vi "TRA server.vi"() -> ()   [LabVIEW 2011]
uses:
  <vilib>/regexp/Match Regular Expression.xnode
panel:
  out "SEND ME TO TRA":string
  in  "Active":bool=TRUE
  out "stopCmd":bool
  out "stopAnswer":string
  out "sema free":bool
  out "Answer Q":refnum<queue>
  out "CmdID":string
  out "in Progress":bool=TRUE
  out "Diode":bool
  in  "STOP":bool
  in  "Tab Control":enum32{"Main", "Config", "Error", "History"}(tab)=enum."Config"
  out "time between two execution":u32
  out "answer":string
  in  "reset array":bool=TRUE
  out "ExecutedCmd":T1(array[cluster])
  out "ConnectArray":T2(array[cluster])
  in  "Picopad Name":string="TRA1"
  in  "Mode GPIB / VISA":bool
  out "NameComment":string
  in  "Port":i32=63430
  out "DevicesConnected":string[][](array[string])
  out "CmdInProgress":T3(array[cluster])
  out "A Q error":errorcluster
  out "tcp error":errorcluster
  out "History":T1(array[cluster])
  out "stopOc":refnum<k4>
  out "semaphore":T4
  out "timer in":u32
  out "Execute time in":u32
  out "Cmd received":string
  # "Server info:"
  # "Don't wire GPIB and VISA on the same time, VISA will be non reliable"
  # "slot3"
  # "slot5"
  # "Slot1"
  # "slot2"
  # "slot4"
  # "connector1"
  # "connector2"
  # "connector3"
  # "connector4"
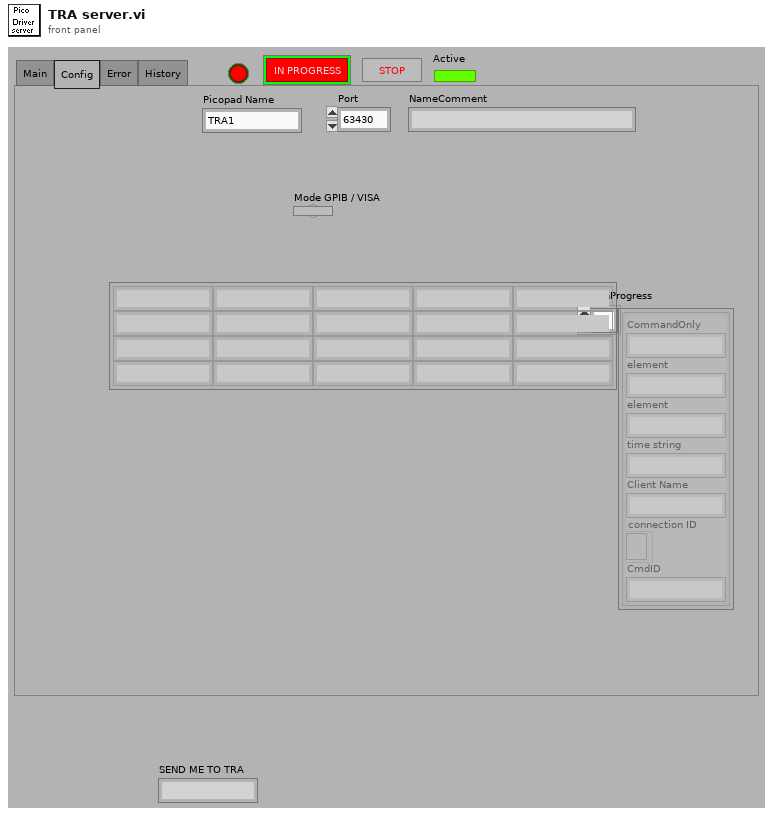
[diagram p1: front panel]
types:
  T1 = cluster{"CommandOnly":string, "status":string, "duration":string, "date":string, "Client Name":string, "connection ID":refnum<k5>, "CmdID":string}[]
  T2 = cluster{"connection ID":refnum<k5>, string, errorcluster}[]
  T3 = cluster{"CommandOnly":string, "element":string, "element":string, "time string":string, "Client Name":string, "connection ID":refnum<k5>, "CmdID":string}[]
  T4 = typedef "Semaphore RefNum" = refnum<k1>
  T5 = cluster{"CommandOnly":string, "element":string, "element":string, "time string":string, "Client Name":string, "connection ID":refnum<k5>, "CmdID":string}
  T6 = cluster{"CommandOnly":string, "status":string, "duration":string, "date":string, "Client Name":string, "connection ID":refnum<k5>, "CmdID":string}
  T7 = cluster{"CommandOnly":string, "status":string, "element":string, "time string":string, "Client Name":string, "connection ID":refnum<k5>, "CmdID":string}
  T8 = cluster{"CommandOnly":string, "status":string, "element":string, "time string":string, "Client Name":string, "connection ID":refnum<k5>, "CmdID":string}[]
  T9 = cluster{"connection ID":refnum<k5>, "remote address":string, "warning out":errorcluster}
  T10 = cluster{"connection ID":refnum<k5>, "remote address":string, "warning out":errorcluster}[]
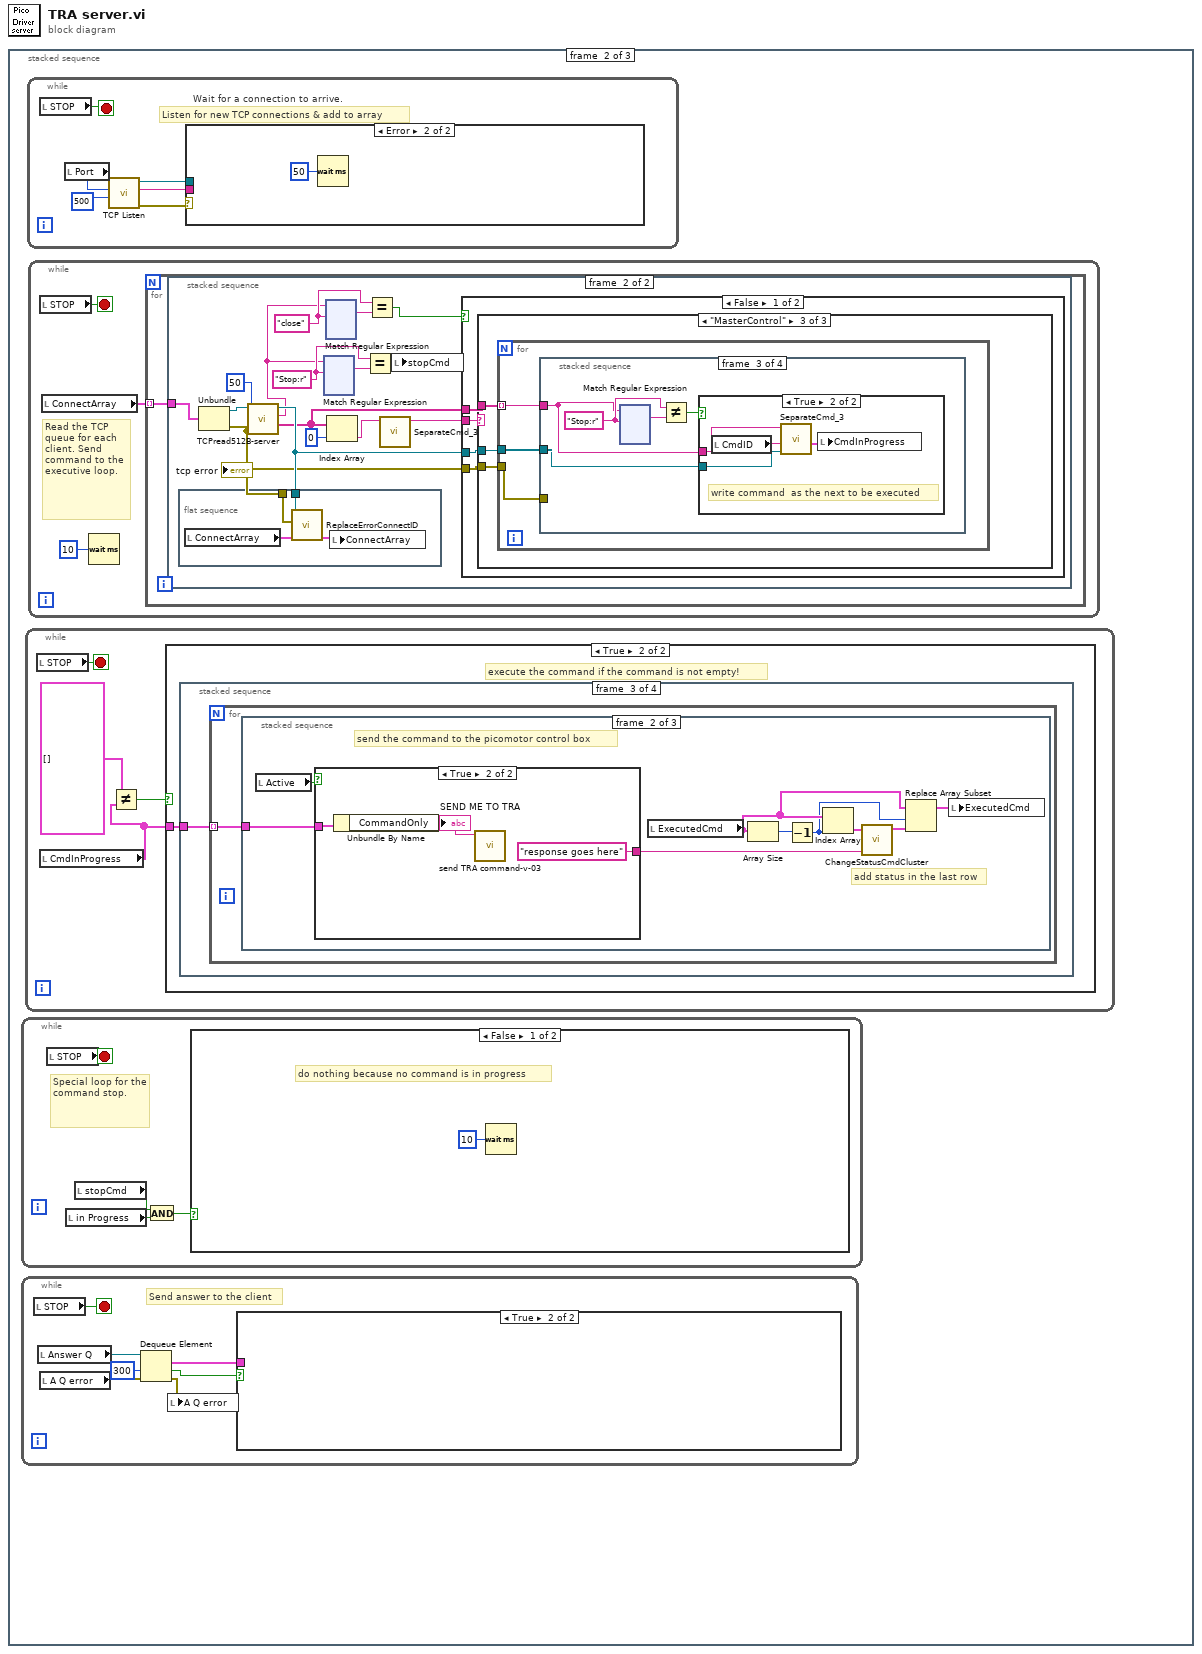
[diagram p0: block diagram]
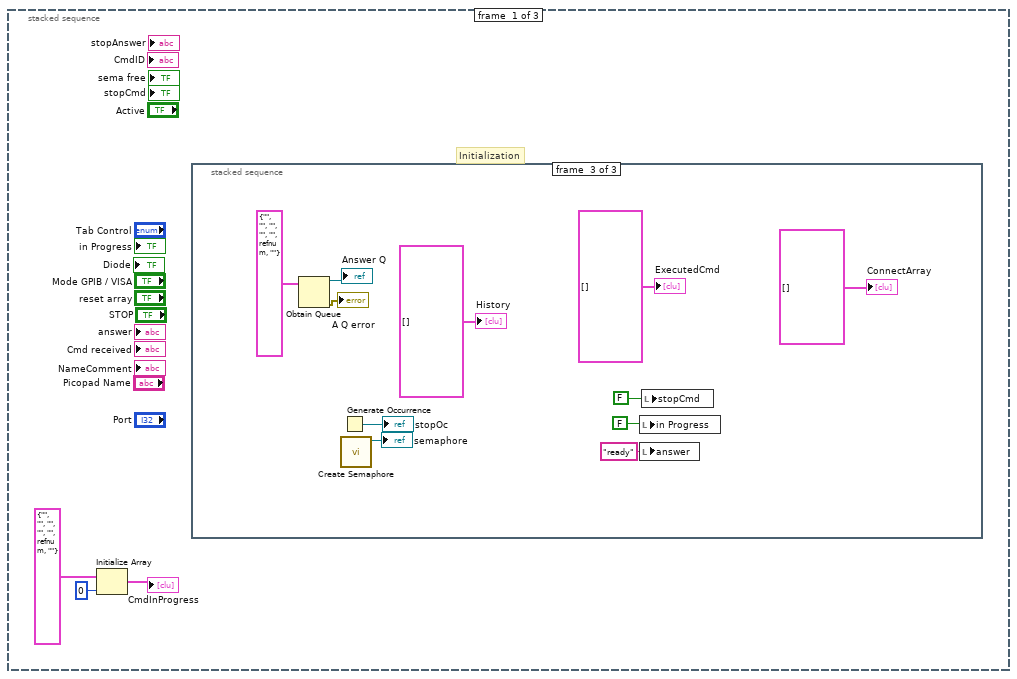
[diagram p2: hidden frame]
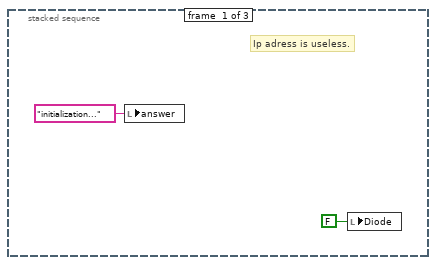
[diagram p3: hidden frame]
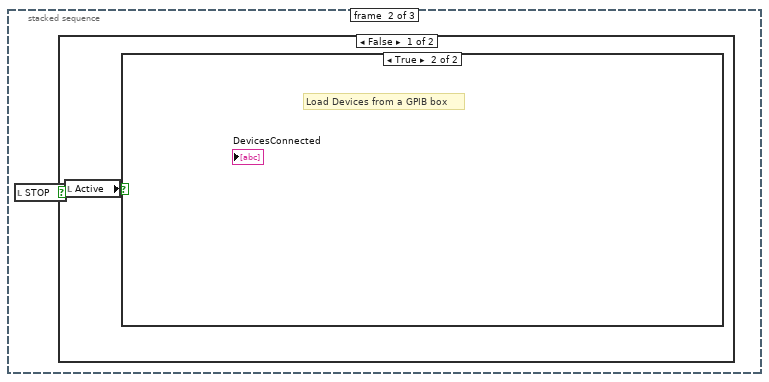
[diagram p4: hidden frame]
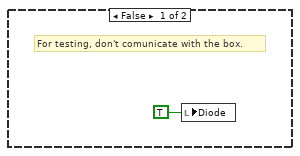
[diagram p5: hidden frame]
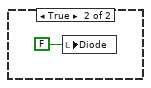
[diagram p6: hidden frame]
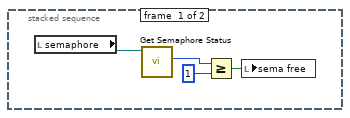
[diagram p7: hidden frame]
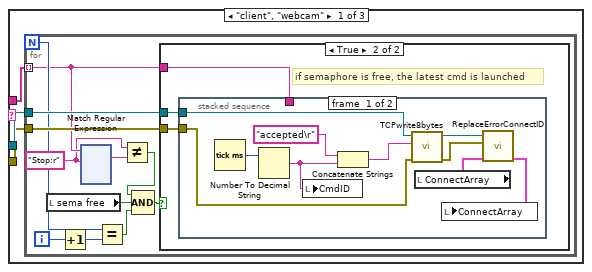
[diagram p8: hidden frame]
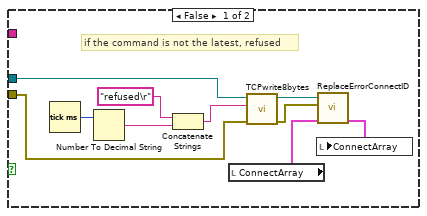
[diagram p9: hidden frame]
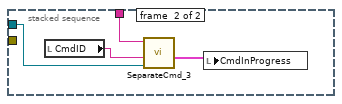
[diagram p10: hidden frame]
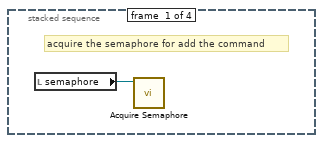
[diagram p12: hidden frame]
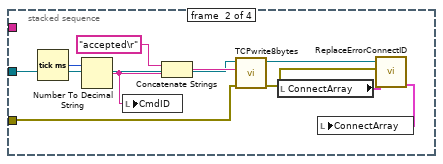
[diagram p13: hidden frame]
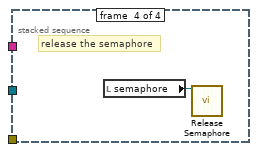
[diagram p15: hidden frame]
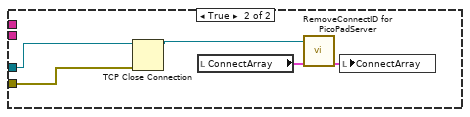
[diagram p16: hidden frame]
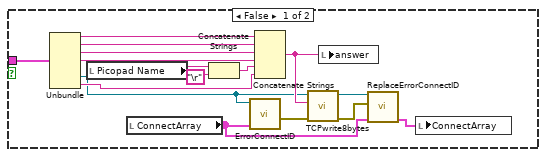
[diagram p17: hidden frame]
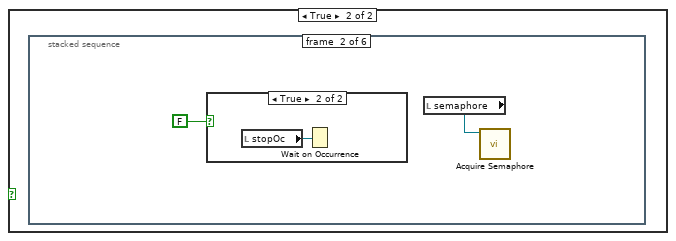
[diagram p18: hidden frame]
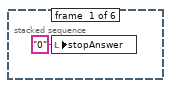
[diagram p19: hidden frame]
diagram:
  n1 = stacked-sequence {
    frame #0 {
      # "Initialization"
      n2 = Initialize Array(T5 {"CommandOnly"="", "element"="", "element"="", "time string"="", "Client Name"="", "connection ID"=refnum, "CmdID"=""} ("CmdInProgress"), 0 ("dimension size")) -> (→"CmdInProgress":T3)
      n3 = stacked-sequence {
        frame #0 {
          # "Ip adress is useless."
          n4 = local write "answer"("initialization..." ("answer")) -> ()
          n5 = local write "Diode"(FALSE ("Diode")) -> ()
        }
        frame #1 {
          n6 = local read "STOP"() -> (w6:bool)
          n7 = case shown="False" w6 {
            frame False {
              n8 = local read "Active"() -> (w7:bool)
              n9 = case shown="True" w7 {
                frame False {
                  # "For testing, don't comunicate with the box."
                  n10 = local write "Diode"(TRUE ("Diode")) -> ()
                }
                frame True {
                  # "Load Devices from a GPIB box"
                }
              }
            }
            frame True {
              n11 = local write "Diode"(FALSE ("Diode")) -> ()
            }
          }
        }
        frame #2 {
          n12 = Obtain Queue(element data type=T5 {"CommandOnly"="", "element"="", "element"="", "time string"="", "Client Name"="", "connection ID"=refnum, "CmdID"=""} ("CmdCluster 2")) -> (queue out=→"Answer Q":refnum<queue>, error out=→"A Q error":errorcluster)  [unwired: 3 in, 2 out]
          n13 = Generate Occurrence() -> (→"stopOc":refnum<k4>)
          n14 = call <vilib>:"Create Semaphore.vi"() -> ("semaphore"=→"semaphore":T4)  [unwired: 2 in, 5 out]
          n15 = local write "in Progress"(FALSE ("in Progress")) -> ()
          n16 = local write "answer"("ready" ("answer")) -> ()
          n17 = local write "stopCmd"(FALSE ("stopCmd")) -> ()
          "ConnectArray" <- T2 []
          "ExecutedCmd" <- T3 []
          "History" <- T3 []
        }
      }
    }
    frame #1 {
      n18 = while {
        stop <- w597 stop-if-true
        # "Special loop for the command stop."
        n19 = local read "STOP"() -> (w597:bool)
        n20 = local read "in Progress"() -> (w596:bool)
        n21 = local read "stopCmd"() -> (w594:bool)
        n22 = And(x=w594, y=w596) -> (x .and. y?=w595:bool)
        n23 = case shown="False" w595 {
          frame False {
            # "do nothing because no command is in progress"
            n24 = Wait (ms)(milliseconds to wait=u32 10) -> ()  [unwired: 1 out]
          }
          frame True {
            n25 = stacked-sequence {
              frame #0 {
                n26 = local write "stopAnswer"("0" ("stopAnswer")) -> ()
              }
              frame #1 {
                n27 = case shown="True" FALSE {
                  frame False {
                  }
                  frame True {
                    n28 = local read "stopOc"() -> (w602:refnum<k4>)
                    n29 = Wait on Occurrence(2:w602) -> ()  [unwired: 3 out]
                  }
                }
                n30 = local read "semaphore"() -> (w600:T4)
                n31 = call <vilib>:"Acquire Semaphore.vi"("semaphore"=w600) -> ()  [unwired: 2 in, 5 out]
              }
              frame #2 {
                # "send answer to the command client"
                # "add status in the last row"
                n32 = local read "stopAnswer"() -> (w604:string)
                n33 = xnode "Match Regular Expression"("input string"=w604, "regular expression"="0" ("y")) -> ("whole match"=w617:string)  [unwired: 2 in, 6 out]
                n34 = local read "ExecutedCmd"() -> (w607:T1)
                n35 = Equal?(x=w617, y="0") -> (x = y?=w618:bool)
                n36 = Select(t="aborted\r", s=w618, f=w604) -> (s? t:f=w609:string)
                n37 = Array Size(array=w607) -> (size(s)=w606:i32)
                n38 = Decrement(x=w606) -> (x-1=w605:i32)
                n39 = Index Array(array=w607, index=w605) -> (element=w611:T6)
                n40 = call "ChangeStatusCmdCluster.vi"("status"=w609, "CmdClusterIN"=w611) -> ("CmdClusterOUT"=w608:T7)  [unwired: 9 out]
                n41 = Replace Array Subset(array=w607, new element=w608, index=w605) -> (w610:T1)
                n42 = local write "ExecutedCmd"(w610) -> ()
                n43 = local read "Answer Q"() -> (w615:refnum<queue>)
                n44 = local read "A Q error"() -> (w614:errorcluster)
                n45 = Enqueue Element(queue=w615, element=w608, error in (no error)=w614) -> (error out=w603:errorcluster)  [unwired: 3 out]
                n46 = local write "A Q error"(w603) -> ()
              }
              frame #3 {
                n47 = local read "ConnectArray"() -> (w731:T2)
                n48 = for {
                  tunnel: w731 -> [w737] mode=indexing
                  tunnel: "A client sent a stop command." -> [w733]
                  n49 = Unbundle(w737) -> ("connection ID"=w736:refnum<k5>, w734:errorcluster)  [unwired: 1 out]
                  n50 = call "TCPwrite8bytes.vi"("Error in"=w734, "Cmd In"=w733, "connection ID in"=w736) -> ("Error out"=w732:errorcluster, "connection ID out"=w735:refnum<k5>)  [unwired: 7 out]
                  n51 = local read "ConnectArray"() -> (w739:T2)
                  n52 = call "ReplaceErrorConnectID.vi"("ConnectArrayIN"=w739, "ErrorIN"=w732, "ConnectID"=w735) -> ("ConnectArrayOUT"=w738:T2)  [unwired: 1 in, 7 out]
                  n53 = local write "ConnectArray"(w738) -> ()
                }
              }
              frame #4 {
                # "aquire the semaphore during 5 seconds, so no command could be execute."
                n54 = local write "Diode"(FALSE ("Diode")) -> ()
                n55 = Wait (ms)(milliseconds to wait=u32 5000) -> ()  [unwired: 1 out]
              }
              frame #5 {
                # "release semaphore"
                n56 = local read "semaphore"() -> (w743:T4)
                n57 = call <vilib>:"Release Semaphore.vi"("semaphore"=w743) -> ()  [unwired: 1 in, 6 out]
                n58 = local write "Diode"(TRUE ("Diode")) -> ()
              }
            }
          }
        }
      }
      n59 = while {
        stop <- w573 stop-if-true
        # "Send answer to the client"
        n60 = local read "STOP"() -> (w573:bool)
        n61 = local read "Answer Q"() -> (w577:refnum<queue>)
        n62 = local read "A Q error"() -> (w575:errorcluster)
        n63 = Dequeue Element(queue=w577, timeout in ms (-1)=300, error in (no error)=w575) -> (element=w576:T5, timed out?=w571:bool, error out=w574:errorcluster)  [unwired: 1 out]
        n64 = local write "A Q error"(w574) -> ()
        n65 = case shown="True" w571 {
          tunnel: w576 -> [w593 _]
          frame False {
            n66 = Unbundle(w593) -> ("CommandOnly"=w592:string, "element"=w591:string, "element"=w590:string, "time string"=w588:string, "connection ID"=w581:refnum<k5>, "CmdID"=w587:string)  [unwired: 1 out]
            n67 = local read "Picopad Name"() -> (w586:string)
            n68 = local read "ConnectArray"() -> (w579:T2)
            n69 = Concatenate Strings(w586, "\r") -> (w585:string)
            n70 = call "ErrorConnectID.vi"("ConnectArrayIN"=w579, "ConnectIDin"=w581) -> ("Error"=w580:errorcluster)  [unwired: 9 out]
            n71 = Concatenate Strings(w592, w591, w590, w588, w585, w587) -> (w589:string)
            n72 = call "TCPwrite8bytes.vi"("Error in"=w580, "Cmd In"=w589, "connection ID in"=w581) -> ("Error out"=w578:errorcluster, "connection ID out"=w582:refnum<k5>)  [unwired: 7 out]
            n73 = local write "answer"(w589) -> ()
            n74 = call "ReplaceErrorConnectID.vi"("ConnectArrayIN"=w579, "ErrorIN"=w578, "ConnectID"=w582) -> ("ConnectArrayOUT"=w583:T2)  [unwired: 1 in, 7 out]
            n75 = local write "ConnectArray"(w583) -> ()
          }
          frame True {
          }
        }
      }
      n76 = while {
        stop <- w747 stop-if-true
        n77 = local read "STOP"() -> (w747:bool)
        n78 = local read "CmdInProgress"() -> (w744:T3)
        n79 = Not Equal?(x=T3 [], y=w744) -> (x != y?=w746:bool)
        n80 = case shown="True" w746 {
          tunnel: w744 -> [_ w749]
          frame False {
            n81 = Wait (ms)(milliseconds to wait=u32 10) -> ()  [unwired: 1 out]
          }
          frame True {
            # "execute the command if the command is not empty!"
            n82 = stacked-sequence {
              tunnel: w749 -> [_ _ w768 _]
              frame #0 {
                # "acquire semaphore"
                n83 = local read "semaphore"() -> (w752:T4)
                n84 = local write "in Progress"(TRUE) -> ()
                n85 = call <vilib>:"Acquire Semaphore.vi"("semaphore"=w752) -> ()  [unwired: 2 in, 5 out]
                n86 = local read "timer in"() -> (w754:u32)
                n87 = Tick Count (ms)() -> (millisecond timer value=w753:u32)
                "Execute time in" <- w753
                n88 = Subtract(x=w753, y=w754) -> (x-y=→"time between two execution":u32)
                n89 = local read "reset array"() -> (w750:bool)
                n90 = case shown="True" w750 {
                  frame False {
                  }
                  frame True {
                    # "reset"
                    n91 = local read "ExecutedCmd"() -> (w758:T1)
                    n92 = Delete From Array(array=w758, length=7) -> (array with subset deleted=w759:T1)  [unwired: 1 in, 1 out]
                    n93 = local write "ExecutedCmd"(w759) -> ()
                    n94 = local write "reset array"(FALSE ("reset array")) -> ()
                  }
                }
              }
              frame #1 {
                n95 = while {
                  stop <- w761 continue-if-true
                  # "Historic of the 10 latest executed commands"
                  n96 = local read "ExecutedCmd"() -> (w762:T1)
                  n97 = Array Size(array=w762) -> (size(s)=w763:i32)
                  n98 = Greater?(x=w763, y=10) -> (0:w761:bool)
                  n99 = case shown="True" w761 {
                    frame False {
                    }
                    frame True {
                      n100 = local read "ExecutedCmd"() -> (w765:T1)
                      n101 = Delete From Array ("delete oldest")(array=w765, length=1, index=0 ("index (row)")) -> (array with subset deleted=w766:T1)  [unwired: 1 out]
                      n102 = local write "ExecutedCmd"(w766) -> ()
                    }
                  }
                }
              }
              frame #2 {
                n103 = for {
                  tunnel: w768 -> [w769] mode=indexing
                  n104 = stacked-sequence {
                    tunnel: w769 -> [w770 w773 _]
                    frame #0 {
                      # "Add the command in progress in the interface"
                      n105 = local read "ExecutedCmd"() -> (w772:T1)
                      n106 = Build Array (concatenate)(w772, w770) -> (w771:T3)
                      n107 = local write "ExecutedCmd"(w771) -> ()
                    }
                    frame #1 {
                      # "add status in the last row"
                      # "send the command to the picomotor control box"
                      n108 = local read "Active"() -> (w774:bool)
                      n109 = case shown="True" w774 {
                        tunnel: [w783 "response goes here" ("time string")] -> w780
                        tunnel: w773 -> [w782 w795]
                        frame False {
                          # "For testing, don't comunicate with the box."
                          n110 = disable-structure shown="Disabled" {
                            disable-tunnel: [w788 w792] -> w783
                            disable-tunnel: w782 -> [w785 _]
                            frame Disabled {
                              n111 = Unbundle By Name(w785) -> ("CommandOnly"=w790:string)
                              n112 = Tick Count (ms)() -> (millisecond timer value=w789:u32)
                              n113 = Decimal String To Number(string=w790) -> (number=w786:i32)  [unwired: 3 out]
                              n114 = Subtract(x=w789, y=w786) -> (x-y=w787:u32)
                              n115 = Number To Decimal String(number=w787) -> (decimal integer string=w788:string)  [unwired: 1 out]
                            }
                            frame Enabled {
                              n116 = Get Date/Time String(want seconds? (F)=TRUE) -> (time string=w792:string)  [unwired: 3 out]
                            }
                          }
                          n117 = Wait (ms)(milliseconds to wait=u32 300) -> ()  [unwired: 1 out]
                        }
                        frame True {
                          n118 = Unbundle By Name(w795) -> ("CommandOnly"=w793:string)
                          "SEND ME TO TRA" <- w793
                          n119 = call "send TRA command-v-03.vi"("command"=w793) -> ()  [unwired: 11 in]
                        }
                      }
                      n120 = local read "ExecutedCmd"() -> (w779:T1)
                      n121 = Array Size(array=w779) -> (size(s)=w776:i32)
                      n122 = Decrement(x=w776) -> (x-1=w775:i32)
                      n123 = Index Array(array=w779, index=w775) -> (element=w781:T6)
                      n124 = call "ChangeStatusCmdCluster.vi"("status"=w780, "CmdClusterIN"=w781) -> ("CmdClusterOUT"=w777:T7)  [unwired: 9 out]
                      n125 = Replace Array Subset(array=w779, new element=w777, index=w775) -> (w778:T1)
                      n126 = local write "ExecutedCmd"(w778) -> ()
                    }
                    frame #2 {
                      # "enqueue the last row"
                      # "add executed time in the command row"
                      n127 = local read "Execute time in"() -> (w811:u32)
                      n128 = Tick Count (ms)() -> (millisecond timer value=w812:u32)
                      "timer in" <- w812
                      n129 = Subtract(x=w812, y=w811) -> (x-y=w810:u32)
                      n130 = local read "ExecutedCmd"() -> (w803:T1)
                      n131 = Number To Decimal String(number=w810) -> (decimal integer string=w805:string)  [unwired: 1 out]
                      n132 = Array Size(array=w803) -> (size(s)=w804:i32)
                      n133 = Decrement(x=w804) -> (x-1=w801:i32)
                      n134 = Concatenate Strings(w805, "\r") -> (w800:string)
                      n135 = Index Array(array=w803, index=w801) -> (element=w806:T6)
                      n136 = call "ChangeExecTimeCmdCluster.vi"("ExecTime"=w800, "CmdClusterIN"=w806) -> ("CmdClusterOUT"=w796:T7)  [unwired: 9 out]
                      n137 = Replace Array Subset(array=w803, new element=w796, index=w801) -> (w802:T1)
                      n138 = local read "History"() -> (w798:T1)
                      n139 = local write "ExecutedCmd"(w802) -> ()
                      n140 = Build Array (concatenate)(w798, w796) -> (w797:T8)
                      n141 = local write "History"(w797) -> ()
                      n142 = local read "A Q error"() -> (w807:errorcluster)
                      n143 = local read "Answer Q"() -> (w809:refnum<queue>)
                      n144 = Enqueue Element(queue=w809, element=w796, error in (no error)=w807) -> (error out=w808:errorcluster)  [unwired: 3 out]
                      n145 = local write "A Q error"(w808) -> ()
                    }
                  }
                }
              }
              frame #3 {
                # "synchronyse interface for stop command"
                # "release semaphore"
                # "clear the command executed"
                n146 = local read "semaphore"() -> (w818:T4)
                n147 = local write "in Progress"(FALSE ("in Progress")) -> ()
                n148 = call <vilib>:"Release Semaphore.vi"("semaphore"=w818) -> ()  [unwired: 1 in, 6 out]
                n149 = Initialize Array(T5 {"CommandOnly"="", "element"="", "element"="", "time string"="", "Client Name"="", "connection ID"=refnum, "CmdID"=""} ("CmdInProgress"), 0 ("dimension size")) -> (w815:T3)
                n150 = local write "CmdInProgress"(w815) -> ()
                n151 = local read "stopOc"() -> (w817:refnum<k4>)
                n152 = Set Occurrence(w817) -> ()
              }
            }
          }
        }
      }
      n153 = while {
        stop <- w821 stop-if-true
        # "Listen for new TCP connections & add to array"
        # "Wait for a connection to arrive."
        n154 = local read "STOP"() -> (w821:bool)
        n155 = local read "Port"() -> (w823:i32)
        n156 = call "TCP Listen.vi"("timeout ms (wait forever: -1)"=500, "port"=w823) -> ("error out"=w819:errorcluster, "remote address"=w820:string, "connection ID"=w822:refnum<k5>)  [unwired: 1 in, 6 out]
        n157 = case shown="Error" w819 {
          selector: w819 -> [w827 _]
          tunnel: w822 -> [w832 _]
          tunnel: w820 -> [w831 _]
          frame No Error {
            w825 = 56 items=["No Error", "Argument Error", "Memory Full", "Out of Zone", "End of File", "File Already Open", "Generic File IO Error", "File Not Found", "File Permission Error", "Disk Full", "Duplicate Path", "Too Many Files Open", "Not Enabled", "Resource File Not Found", "Cannot Add Resource", "Resource Not Found", "Image Not Found", "Image Memory Error", "Pen Does Not Exist", "Config Bad Type", "Config Token Not Found", "Config Parse Error", "Config Memory Error", "Bad External Code Format", "Bad External Code Offset", "External Code Not Present", "Null Window", "Destroy Window Mixup", "Null Menu", "Print Aborted", "Bad Print Record", "Print Driver Error", "Windows Error During Print", "Memory Error During Print", "Print Dialog Error", "Generic Print Error", "Invalid Device Refnum", "Device Not Found", "Device Parameter Error", "Device Unit Error", "Can't Open Device", "Device Call Aborted", "Generic Error", "Cancelled By User", "Object ID Too Low", "Object ID Too High", "Object Not In Heap", "Unknown Heap", "Bad DefProc ID", "DefProc Not In Table", "Message Out Of Range", "Null Method", "Unknown Message", "Manager Call Not Supported", "Bad address", "Connection In progress", "Connection timed out", "Connection is already in progress", "Network attribute not supported", "Network error", "Address in use", "System out of memory", "Connection aborted", "Connection refused", "Connection is not connected", "Connection is already connected", "Connection closed", "Initialize error (interapplication manager)", "Bad occurrence", "Wait on unbound occurrence handler", "Occurrence queue overflow", "Bad path", "Semaphore not signaled", "Unrecognized type (interapplication manager)"] ("1st Error to Convert")
            n158 = call <vilib>:"Error to Warning.vi"("1st Error to Convert"=w825, "error in"=w827) -> ("warning out"=w826:errorcluster)  [unwired: 3 in, 10 out]
            n159 = Bundle("connection ID"=w832, "remote address"=w831, "warning out"=w826) -> (w830:T9)  [unwired: 1 out]
            n160 = local read "ConnectArray"() -> (w829:T2)
            n161 = Build Array (concatenate)(w829, w830) -> (w828:T10)
            n162 = local write "ConnectArray"(w828) -> ()
          }
          frame Error {
            n163 = Wait (ms)(milliseconds to wait=u32 50) -> ()  [unwired: 1 out]
          }
        }
      }
      n164 = while {
        stop <- w23 stop-if-true
        # "Read the TCP queue for each client. Send command to the executive loop."
        n165 = local read "STOP"() -> (w23:bool)
        n166 = local read "ConnectArray"() -> (w21:T2)
        n167 = Wait (ms)(milliseconds to wait=u32 10) -> ()  [unwired: 1 out]
        n168 = for {
          tunnel: w21 -> [w24] mode=indexing
          n169 = stacked-sequence {
            tunnel: w24 -> [_ w42]
            frame #0 {
              n170 = local read "semaphore"() -> (w28:T4)
              n171 = call <vilib>:"Get Semaphore Status.vi"("semaphore"=w28) -> ("# available"=w25:i32)  [unwired: 1 in, 9 out]
              n172 = Greater Or Equal?(x=w25, y=1) -> (x >= y?=w26:bool)
              n173 = local write "sema free"(w26) -> ()
            }
            frame #1 {
              w32 = "close"
              w35 = "Stop:r"
              n174 = flat-sequence {
                tunnel: w39 -> [w570]
                tunnel: w33 -> [w567]
                frame #0 {
                  n175 = local read "ConnectArray"() -> (w569:T2)
                  n176 = call "ReplaceErrorConnectID.vi"("ConnectArrayIN"=w569, "ErrorIN"=w567, "ConnectID"=w570) -> ("ConnectArrayOUT"=w568:T2)  [unwired: 8 out]
                  n177 = local write "ConnectArray"(w568) -> ()
                }
              }
              n178 = Unbundle(w42) -> ("connection ID"=w43:refnum<k5>, w33:errorcluster)  [unwired: 1 out]
              "tcp error" <- w33
              n179 = call "TCPread512B-server.vi"("Error in"=w33, "timeout ms (25000)"=50, "connection ID in"=w43) -> ("Array"=w37:string[], "string out"=w30:string, "connection ID out"=w39:refnum<k5>)  [unwired: 6 out]
              n180 = xnode "Match Regular Expression"("input string"=w30, "regular expression"=w35) -> ("whole match"=w36:string)  [unwired: 2 in, 6 out]
              n181 = xnode "Match Regular Expression"("input string"=w30, "regular expression"=w32) -> ("whole match"=w31:string)  [unwired: 2 in, 6 out]
              n182 = Index Array(array=w37, index=0) -> (element=w38:string)
              n183 = Equal?(x=w35, y=w36) -> (x = y?=w34:bool)
              n184 = Equal?(x=w32, y=w31) -> (x = y?=w29:bool)
              n185 = call "SeparateCmd_3.vi"("command received"=w38) -> ("Client Name"=w40:string)  [unwired: 2 in, 8 out]
              n186 = local write "stopCmd"(w34) -> ()
              n187 = case shown="False" w29 {
                tunnel: w40 -> [w48 _]
                tunnel: w39 -> [w47 w344]
                tunnel: w37 -> [w46 _]
                tunnel: w33 -> [w45 w343]
                frame False {
                  n188 = case shown="\"MasterControl\"" w48 {
                    tunnel: w47 -> [w50 _ w204]
                    tunnel: w45 -> [w49 _ w203]
                    tunnel: w46 -> [w51 _ w202]
                    frame "client", "webcam" {
                      n189 = for {
                        N -> [w58]
                        tunnel: w51 -> [w54] mode=indexing
                        tunnel: w50 -> [w63]
                        tunnel: w49 -> [w62]
                        i -> [w59]
                        w52 = "Stop:r"
                        n190 = local read "sema free"() -> (w60:bool)
                        n191 = Increment(x=w59) -> (x+1=w56:i32)
                        n192 = xnode "Match Regular Expression"("input string"=w54, "regular expression"=w52) -> ("whole match"=w55:string)  [unwired: 3 in, 5 out]
                        n193 = Equal?(x=w58, y=w56) -> (x = y?=w57:bool)
                        n194 = Not Equal?(x=w52, y=w55) -> (x != y?=w53:bool)
                        n195 = Compound Arithmetic op=AND(w53, w60, w57) -> (w61:bool)
                        n196 = case shown="True" w61 {
                          tunnel: w54 -> [_ w185]
                          tunnel: w63 -> [w179 w187]
                          tunnel: w62 -> [w178 w186]
                          frame False {
                            # "if the command is not the latest, refused"
                            n197 = Tick Count (ms)() -> (millisecond timer value=w184:u32)
                            n198 = Number To Decimal String(number=w184) -> (decimal integer string=w181:string)  [unwired: 1 out]
                            n199 = Concatenate Strings("refused\r" ("Command status"), w181) -> (w180:string)
                            n200 = local read "ConnectArray"() -> (w177:T2)
                            n201 = call "TCPwrite8bytes.vi"("Error in"=w178, "Cmd In"=w180, "connection ID in"=w179) -> ("Error out"=w175:errorcluster, "connection ID out"=w182:refnum<k5>)  [unwired: 7 out]
                            n202 = call "ReplaceErrorConnectID.vi"("ConnectArrayIN"=w177, "ErrorIN"=w175, "ConnectID"=w182) -> ("ConnectArrayOUT"=w176:T2)  [unwired: 1 in, 7 out]
                            n203 = local write "ConnectArray"(w176) -> ()
                          }
                          frame True {
                            # "if semaphore is free, the latest cmd is launched"
                            n204 = stacked-sequence {
                              tunnel: w187 -> [w192 w200]
                              tunnel: w186 -> [w191 _]
                              tunnel: w185 -> [_ w201]
                              frame #0 {
                                n205 = Tick Count (ms)() -> (millisecond timer value=w197:u32)
                                n206 = Number To Decimal String(number=w197) -> (decimal integer string=w193:string)  [unwired: 1 out]
                                n207 = local write "CmdID"(w193) -> ()
                                n208 = Concatenate Strings("accepted\r" ("Command status"), w193) -> (w195:string)
                                n209 = call "TCPwrite8bytes.vi"("Error in"=w191, "Cmd In"=w195, "connection ID in"=w192) -> ("Error out"=w188:errorcluster, "connection ID out"=w194:refnum<k5>)  [unwired: 7 out]
                                n210 = local read "ConnectArray"() -> (w189:T2)
                                n211 = call "ReplaceErrorConnectID.vi"("ConnectArrayIN"=w189, "ErrorIN"=w188, "ConnectID"=w194) -> ("ConnectArrayOUT"=w190:T2)  [unwired: 1 in, 7 out]
                                n212 = local write "ConnectArray"(w190) -> ()
                              }
                              frame #1 {
                                n213 = local read "CmdID"() -> (w199:string)
                                n214 = call "SeparateCmd_3.vi"("connection ID"=w200, "CmdID"=w199, "command received"=w201) -> ("CmdInProgress"=w198:T3)  [unwired: 8 out]
                                n215 = local write "CmdInProgress"(w198) -> ()
                              }
                            }
                          }
                        }
                      }
                    }
                    frame Default {
                    }
                    frame "MasterControl" {
                      n216 = for {
                        tunnel: w204 -> [w207]
                        tunnel: w203 -> [w206]
                        tunnel: w202 -> [w205] mode=indexing
                        n217 = stacked-sequence {
                          tunnel: w207 -> [_ w215 w223 _]
                          tunnel: w206 -> [_ w214 _ _]
                          tunnel: w205 -> [_ _ w220 _]
                          frame #0 {
                            # "acquire the semaphore for add the command"
                            n218 = local read "semaphore"() -> (w208:T4)
                            n219 = call <vilib>:"Acquire Semaphore.vi"("semaphore"=w208) -> ()  [unwired: 2 in, 5 out]
                          }
                          frame #1 {
                            n220 = Tick Count (ms)() -> (millisecond timer value=w218:u32)
                            n221 = Number To Decimal String(number=w218) -> (decimal integer string=w210:string)  [unwired: 1 out]
                            n222 = local write "CmdID"(w210) -> ()
                            n223 = Concatenate Strings("accepted\r" ("Command status"), w210) -> (w216:string)
                            n224 = call "TCPwrite8bytes.vi"("Error in"=w214, "Cmd In"=w216, "connection ID in"=w215) -> ("Error out"=w209:errorcluster, "connection ID out"=w211:refnum<k5>)  [unwired: 7 out]
                            n225 = local read "ConnectArray"() -> (w212:T2)
                            n226 = call "ReplaceErrorConnectID.vi"("ConnectArrayIN"=w212, "ErrorIN"=w209, "ConnectID"=w211) -> ("ConnectArrayOUT"=w213:T2)  [unwired: 1 in, 7 out]
                            n227 = local write "ConnectArray"(w213) -> ()
                          }
                          frame #2 {
                            w221 = "Stop:r"
                            n228 = xnode "Match Regular Expression"("input string"=w220, "regular expression"=w221) -> ("whole match"=w222:string)  [unwired: 3 in, 5 out]
                            n229 = Not Equal?(x=w221, y=w222) -> (x != y?=w219:bool)
                            n230 = case shown="True" w219 {
                              tunnel: w223 -> [_ w227]
                              tunnel: w220 -> [_ w225]
                              frame False {
                                # "stop commamds are processed by a special loop."
                                # "if it's a stop command, do nothing."
                              }
                              frame True {
                                # "write command  as the next to be executed"
                                n231 = local read "CmdID"() -> (w226:string)
                                n232 = call "SeparateCmd_3.vi"("connection ID"=w227, "CmdID"=w226, "command received"=w225) -> ("CmdInProgress"=w224:T3)  [unwired: 8 out]
                                n233 = local write "CmdInProgress"(w224) -> ()
                              }
                            }
                          }
                          frame #3 {
                            # "release the semaphore"
                            n234 = local read "semaphore"() -> (w339:T4)
                            n235 = call <vilib>:"Release Semaphore.vi"("semaphore"=w339) -> ()  [unwired: 1 in, 6 out]
                          }
                        }
                      }
                    }
                  }
                }
                frame True {
                  n236 = TCP Close Connection(connection ID=w344, error in (no error)=w343) -> (connection ID out=w340:refnum<k5>)  [unwired: 2 out]
                  n237 = local read "ConnectArray"() -> (w341:T2)
                  n238 = call "RemoveConnectID for PicoPadServer.vi"("ConnectArrayIN"=w341, "ConnectID"=w340) -> ("ConnectArrayOUT"=w342:T2)  [unwired: 9 out]
                  n239 = local write "ConnectArray"(w342) -> ()
                }
              }
            }
          }
        }
      }
    }
    frame #2 {
      # "Close the connection to the box and clear devices list"
      n240 = local write "answer"("stopping" ("answer")) -> ()
      n241 = local write "STOP"(FALSE ("STOP")) -> ()
    }
  }
